vi "Dpc Set Pin State.vi"(7 "ptrid":u16, 8 "error in (no error)":errorcluster, 9 "erc":i32, 10 "fsState":u32, 11 "hif":u32) -> (0 "error out":errorcluster, 1 "erc out":i32, 2 "function return":i32, 3 "hif out":u32, 5 "ptrid out":u16)   [LabVIEW 2011, in "LVH-Adept.lvlib" / "DPCUTIL.lvlib"]
doc: "DPCAPI BOOL DpcSetPinState(HANDLE hif, DWORD fsState, ERC * erc, TRID * ptrid);"
uses:
  DPCUTIL.lvlib
  Resources/dpcutil.dll
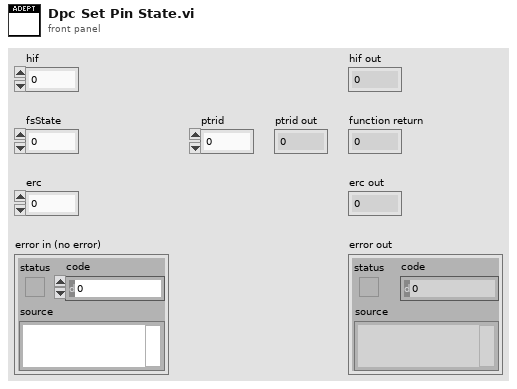
[diagram p1: front panel]
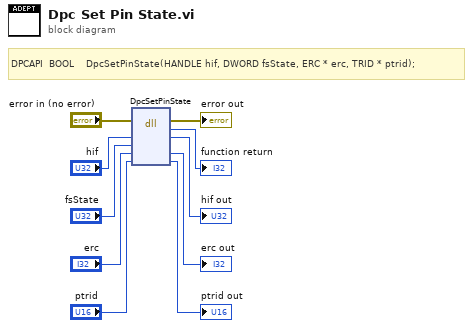
[diagram p0: block diagram]
diagram:
  # "DPCAPI  BOOL    DpcSetPinState(HANDLE hif, DWORD fsState, ERC * erc, TRID * ptrid);"
  n1 = dll-call lib="C:/github/labviewhacker/LVH-Adept/LabVIEW/vi.lib/LabVIEW Hacker/Adept/Private/Resources/dpcutil.*" fn="DpcSetPinState"(error in="error in (no error)", "hif"="hif", "fsState"="fsState", "erc"="erc", "ptrid"="ptrid") -> (error out=→"error out":errorcluster, →"function return":i32, "hif"=→"hif out":u32, "erc"=→"erc out":i32, "ptrid"=→"ptrid out":u16)  [unwired: 3 in, 1 out]
